vi "Init.vi"(8 "error in (no error)":errorcluster, 9 "Child":refnum<class "CConfig Object.lvclass">, 10 "Data":string[](array[string])) -> (0 "error out":errorcluster, 3 "Composite Object out":refnum<class "CConfig Object.lvclass">)   [LabVIEW 2013, in "CConfig Object.lvclass"]
doc: "Copyright 2018, Carya Automatisering, Wiebe Walstra."
uses:
  CConfig Object.lvclass
  CConfig Object.lvclass/CConfig Object.ctl
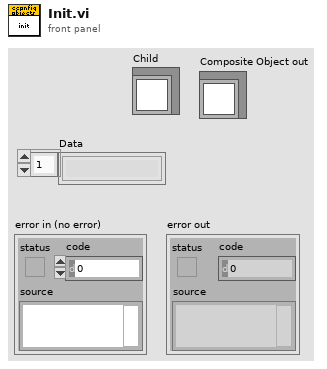
[diagram p1: front panel]
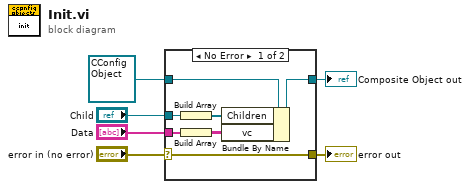
[diagram p0: block diagram]
diagram:
  n1 = case shown="No Error" "error in (no error)" {
    selector: "error in (no error)" -> [w13 w15]
    tunnel: [w13 w15] -> w5
    tunnel: [w11 w14] -> w4
    tunnel: refnum<class "CConfig Object.lvclass"> refnum ("Composite Object in") -> [w12 w14]
    tunnel: "Data" -> [w8 _]
    tunnel: "Child" -> [w10 _]
    frame No Error {
      n2 = Build Array(w10) -> (w9:refnum<class "CConfig Object.lvclass">[])
      n3 = Build Array(w8) -> (w7:string[][])
      n4 = Bundle By Name(cluster=w12, "Children"=w9, "vc"=w7) -> (w11:refnum<class "CConfig Object.lvclass">)
    }
    frame Error {
    }
  }
  "error out" <- w5
  "Composite Object out" <- w4
